vi "AdcCalc.vi"(8 "error in (no error)":errorcluster, 10 "Array":u32[](array[numeric]), 11 "BME680 in":refnum<class "BME680.lvclass">) -> (0 "error out":errorcluster, 1 "Adc Hum":u32, 2 "Adc Temp":u32, 3 "BME680 out":refnum<class "BME680.lvclass">, 5 "Adc Pres":u32)   [LabVIEW 2022 SP3, in "BME680.lvlib" / "BME680.lvclass"]
uses:
  BME680.lvclass
  BME680.lvclass/BME680.ctl
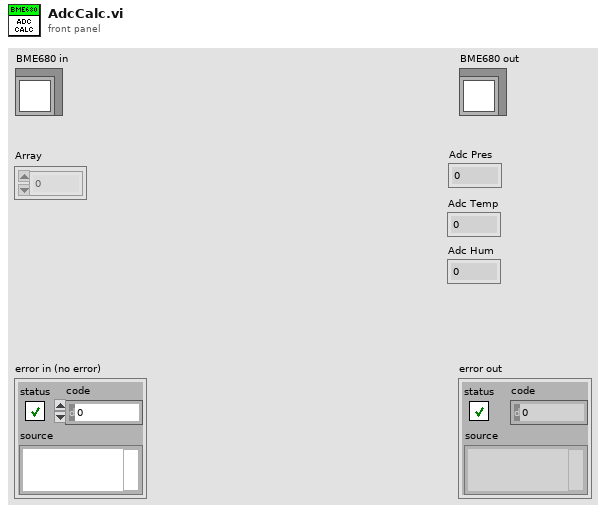
[diagram p1: front panel]
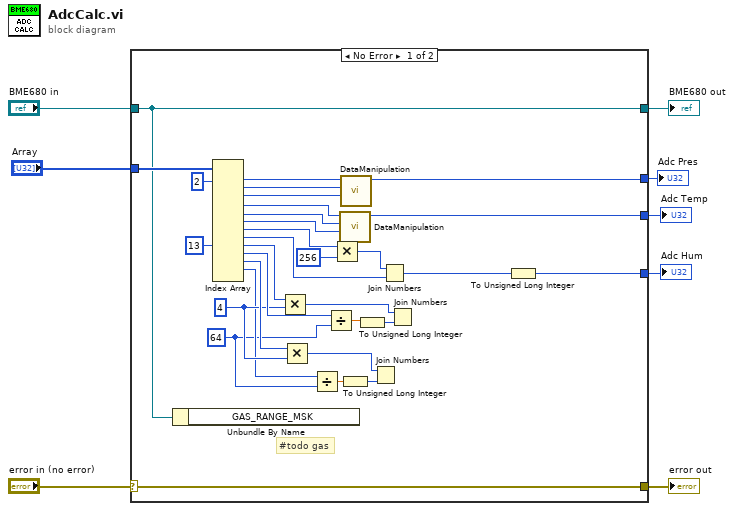
[diagram p0: block diagram]
diagram:
  n1 = case shown="No Error" "error in (no error)" {
    selector: "error in (no error)" -> [w39 w41]
    tunnel: [w39 w41] -> w7
    tunnel: [w13 w40] -> w5
    tunnel: "BME680 in" -> [w13 w40]
    tunnel: "Array" -> [w38 _]
    tunnel: [w9 _] -> w1
    tunnel: [w12 _] -> w2
    tunnel: [w11 _] -> w3
    frame No Error {
      w20 = 64
      w22 = 4
      # "#todo gas"
      n2 = Unbundle By Name(w13) -> ()  [unwired: 1 out]
      n3 = Index Array(array=w38, index #1=2 ("index"), index #9=13 ("index")) -> (element #1=w36:u32, element #2=w35:u32, element #3=w34:u32, element #4=w33:u32, element #5=w32:u32, element #6=w31:u32, element #7=w29:u32, element #8=w27:u32, element #9=w25:u32, element #10=w24:u32, element #11=w23:u32, element #12=w21:u32)  [unwired: 11 in, 1 out]
      n4 = Multiply(x=w25, y=w22) -> (x*y=w16:u32)
      n5 = Multiply(x=w23, y=w22) -> (x*y=w14:u32)
      n6 = Divide(x=w21, y=w20) -> (x/y=w18:dbl)
      n7 = Divide(x=w24, y=w20) -> (x/y=w19:dbl)
      n8 = Multiply(x=w29, y=256) -> (x*y=w28:u32)
      n9 = call "DataManipulation.vi"("y3"=w31, "y 2"=w32, "y"=w33) -> ("Data out"=w12:u32)  [unwired: 8 in]
      n10 = To Unsigned Long Integer(number=w18) -> (unsigned 32bit integer=w15:u32)
      n11 = call "DataManipulation.vi"("y3"=w34, "y 2"=w35, "y"=w36) -> ("Data out"=w11:u32)  [unwired: 8 in]
      n12 = To Unsigned Long Integer(number=w19) -> (unsigned 32bit integer=w17:u32)
      n13 = Join Numbers(hi=w14, lo=w15) -> ()  [unwired: 1 out]
      n14 = Join Numbers(hi=w28, lo=w27) -> ((hi.lo)=w10:u64)
      n15 = Join Numbers(hi=w16, lo=w17) -> ()  [unwired: 1 out]
      n16 = To Unsigned Long Integer(number=w10) -> (unsigned 32bit integer=w9:u32)
    }
    frame Error {
    }
  }
  "error out" <- w7
  "BME680 out" <- w5
  "Adc Pres" <- w3
  "Adc Temp" <- w2
  "Adc Hum" <- w1
